vi "FTW-Ether-NewTagConnection.vi"(5 "Tag Address":string, 11 "error in":errorcluster) -> (4 "Tag Connection":refnum<class "FTW-ActorConnector.lvclass">, 15 "error out":errorcluster)   [LabVIEW 2015, in "FTW-Ether.lvclass"]
uses:
  FTW-Ether.lvclass
  Connector/FTW-ActorConnector.lvclass
  FTW-Ether-Instance.vi
panel:
  # "Inputs"
  # "Outputs"
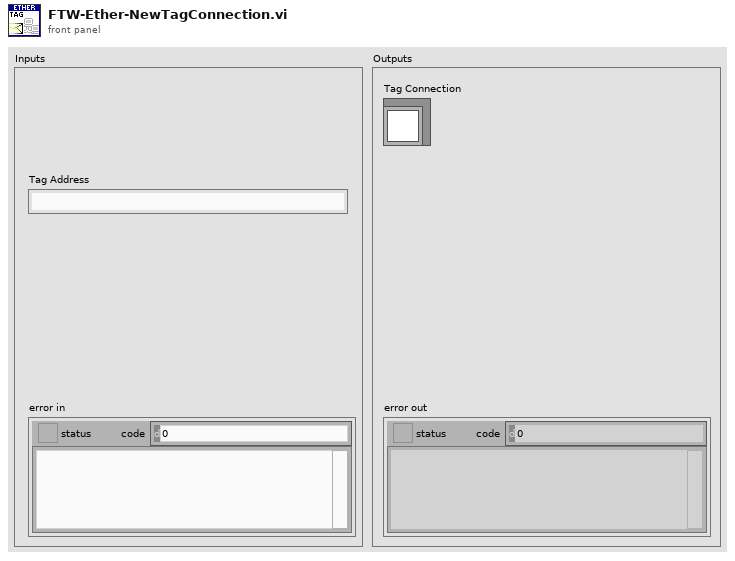
[diagram p1: front panel]
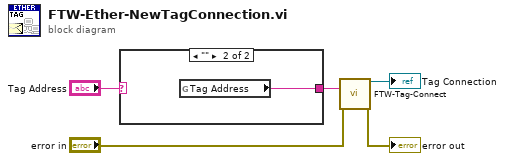
[diagram p0: block diagram]
diagram:
  n1 = case shown="\"\"" "Tag Address" {
    selector: "Tag Address" -> [w6 _]
    tunnel: [w6 w7] -> w2
    frame Default {
    }
    frame "" {
      n2 = global read "FTW-Ether-Instance.vi" "Tag Address"() -> (w7:string)
    }
  }
  n3 = call "FTW-Tag-Connect.vi"("Tag Address"=w2, "error in"="error in") -> ("FTW Tag Connector"=→"Tag Connection":refnum<class "FTW-ActorConnector.lvclass">, "error out"=→"error out":errorcluster)  [unwired: 12 in]
